vi "AlignDUT_Striptest.vi"(9 "New Sensor?":bool, 10 "ProbeStationControl in":refnum<class "ProbeStationControl.lvclass">) -> (2 "ProbeStationControl in 3":refnum<class "ProbeStationControl.lvclass">)   [LabVIEW 2019]
uses:
  itk-strip-sensor-qc/LabVIEW 2019/InstrControl/ProbeStationControl/ProbeStationControl.lvclass
  <vilib>/userDefined/High Color/IMAQdx.ctl
  <vilib>/vision/driver/NI_Vision_Acquisition_Software.lvlib
  <vilib>/vision/NI_Vision_Development_Module.lvlib
panel:
  out "Average Length Between Fiducials":dbl format="%0.2f"
  in  "Number of Iterations":i32=1
  in  "Sensor Type":string(combo)="ATLAS12R0"
  in  "Second Move OK?":bool
  in  "Second Fiducial OK?":bool
  in  "Second Fiducial in View?":bool
  in  "First Move OK?":bool
  in  "First Fiducial OK?":bool
  out "Pattern Matched Image":T1(plugin-control) caption="Template Image"
  out "Image Out":T1(plugin-control)
  in  "Fiducial 1":bool
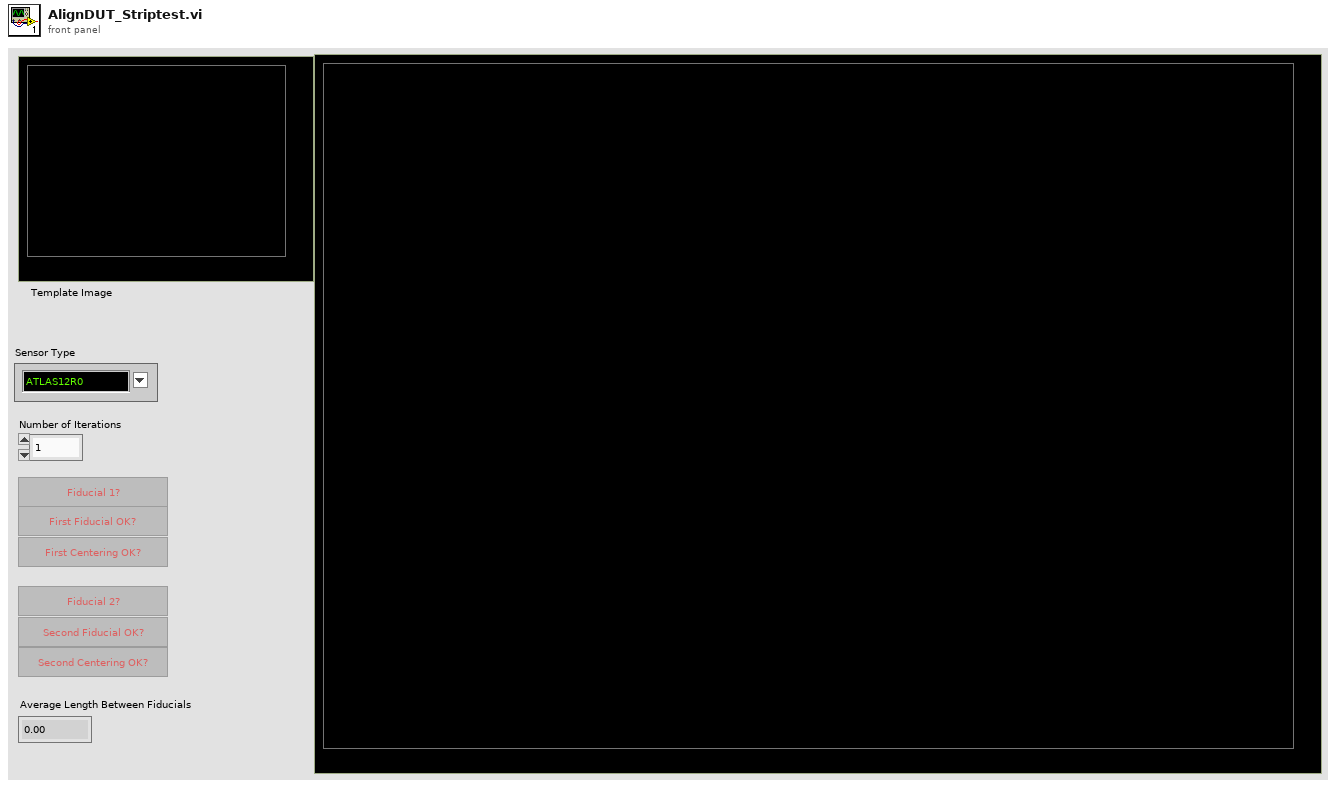
[diagram p1: front panel]
types:
  T1 = typedef "IMAQ Image.ctl" = refnum<image>
  T2 = typedef "IMAQdx.ctl" = refnum<k21>
  T3 = enum8{"Enabled", "Disabled", "Disabled and Grayed Out"}
  T4 = typedef "Image Type" = u32
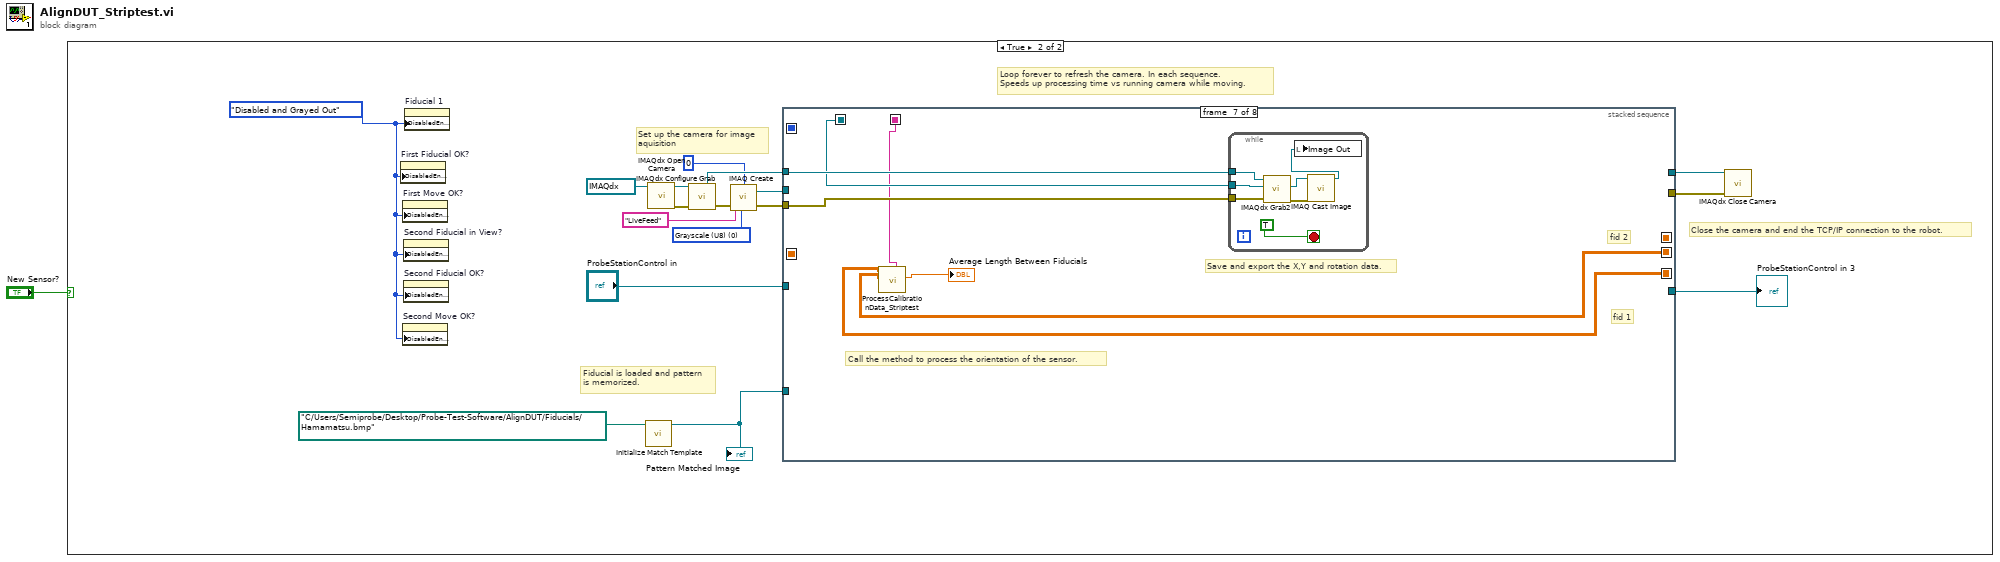
[diagram p0: block diagram]
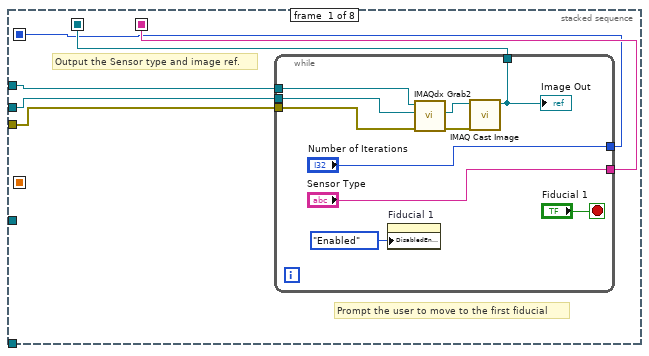
[diagram p3: hidden frame]
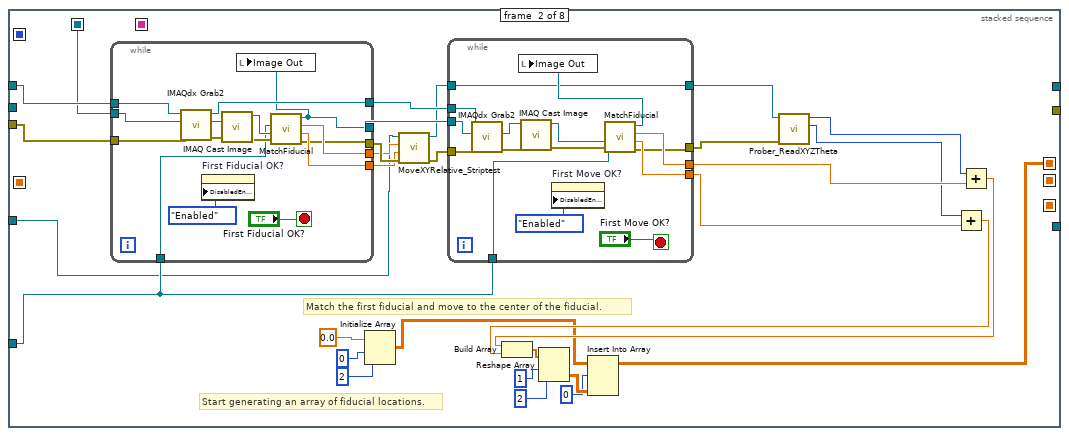
[diagram p4: hidden frame]
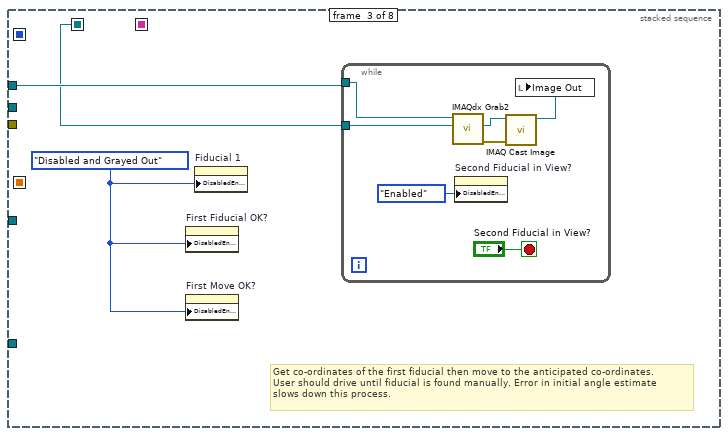
[diagram p5: hidden frame]
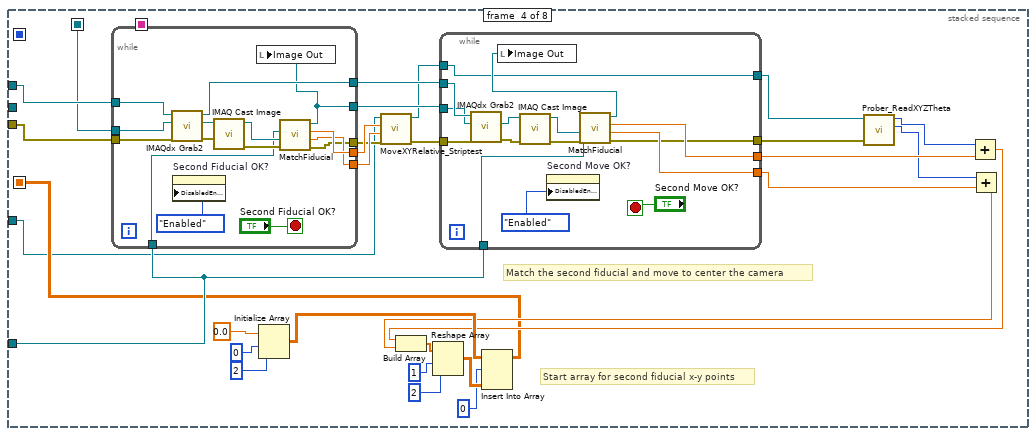
[diagram p6: hidden frame]
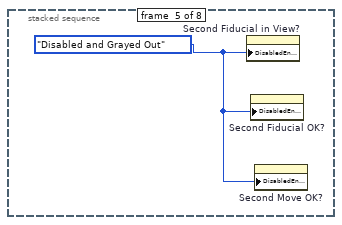
[diagram p7: hidden frame]
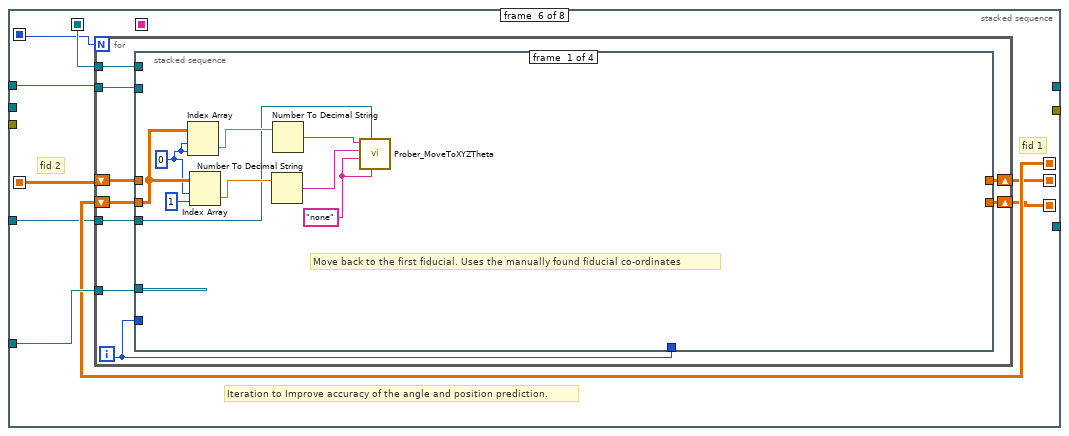
[diagram p8: hidden frame]
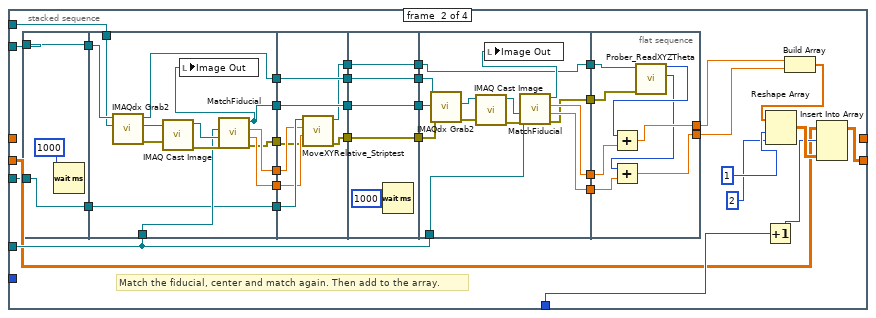
[diagram p9: hidden frame]
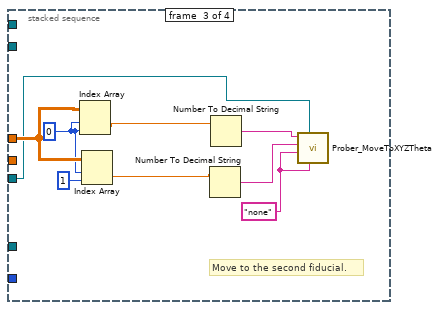
[diagram p10: hidden frame]
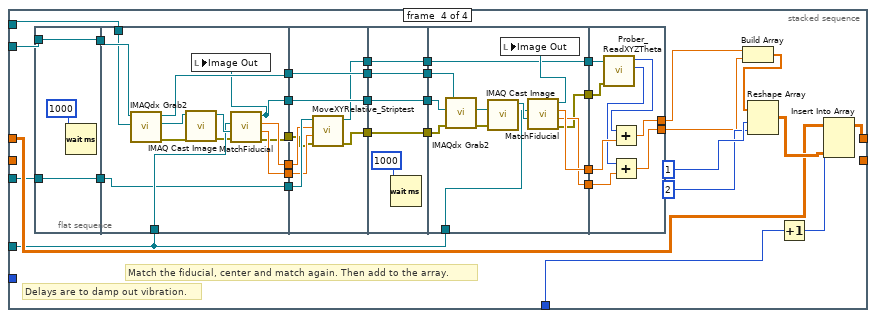
[diagram p11: hidden frame]
diagram:
  n1 = case shown="True" "New Sensor?" {
    frame False {
    }
    frame True {
      w5 = T3."Disabled and Grayed Out" ("Disabled")
      w7 = T4 0 items=["Grayscale (U8)", "Grayscale (I16)", "Grayscale (SGL)", "Complex (CSG)", "RGB (U32)", "HSL (U32)", "RGB (U64)", "Grayscale (U16)"] ("Image Type")
      # "Close the camera and end the TCP/IP connection to the robot."
      # "Fiducial is loaded and pattern\nis memorized."
      # "Loop forever to refresh the camera. In each sequence. \nSpeeds up processing time vs running camera while moving."
      # "Set up the camera for image \naquisition"
      n2 = property on="First Fiducial OK?" class="Bool"("DisabledEnum"=w5) -> ()  [unwired: 2 in, 2 out]
      n3 = property on="First Move OK?" class="Bool"("DisabledEnum"=w5) -> ()  [unwired: 2 in, 2 out]
      n4 = property on="Second Move OK?" class="Bool"("DisabledEnum"=w5) -> ()  [unwired: 2 in, 2 out]
      n5 = property on="Second Fiducial in View?" class="Bool"("DisabledEnum"=w5) -> ()  [unwired: 2 in, 2 out]
      n6 = property on="Second Fiducial OK?" class="Bool"("DisabledEnum"=w5) -> ()  [unwired: 2 in, 2 out]
      n7 = property on="Fiducial 1" class="Bool"("DisabledEnum"=w5) -> ()  [unwired: 2 in, 2 out]
      n8 = call "Initialize Match Template.vi"("base path"=path "C:/Users/Semiprobe/Desktop/Probe-Test-Software/AlignDUT/Fiducials/Hamamatsu.bmp") -> ("Pattern Matched Image"=w10:T1)  [unwired: 10 in]
      "Pattern Matched Image" <- w10
      n9 = call <vilib>:"IMAQdx Open Camera.vi"("Session In"=T2 "cam0") -> ("error out"=w16:errorcluster, "Session Out"=w17:T2)  [unwired: 9 in]
      n10 = call <vilib>:"IMAQdx Configure Grab.vi"("error in"=w16, "Session In"=w17) -> ("error out"=w14:errorcluster, "Session Out"=w13:T2)  [unwired: 8 in]
      n11 = call "IMAQ Create"("Border Size"=0, "Image Name"="LiveFeed", "Image Type"=w7, "error in (no error)"=w14) -> ("New Image"=w12:T1, "error out"=w11:errorcluster)  [unwired: 1 in]
      n12 = stacked-sequence {
        seq-local: [_ _ _ w115 _ _ _ _] -> [_ _ _ _ _ w174 _ _]
        seq-local: [w21 _ _ _ _ _ _ _] -> [_ w59 w96 w130 _ w173 w373 _]
        seq-local: [_ w46 _ _ _ _ _ _] -> [_ _ _ _ _ w170 _ _]
        seq-local: [_ _ _ _ _ w168 _ _] -> [_ _ _ _ _ _ w371 _]
        seq-local: [_ _ _ _ _ w169 _ _] -> [_ _ _ _ _ _ w372 _]
        seq-local: [w20 _ _ _ _ _ _ _] -> [_ _ _ _ _ _ w370 _]
        seq-local: [w19 _ _ _ _ _ _ _] -> [_ _ _ _ _ w167 _ _]
        tunnel: w13 -> [w24 w64 w97 w131 _ w172 w375 w384]
        tunnel: w12 -> [w23 _ _ _ _ _ _ _]
        tunnel: w11 -> [w22 w61 _ w133 _ _ w374 w385]
        tunnel: w10 -> [_ w62 _ w132 _ w171 _ _]
        tunnel: [_ _ _ _ _ _ _ w385] -> w9
        tunnel: [_ _ _ _ _ _ _ w384] -> w8
        tunnel: "ProbeStationControl in" -> [_ w41 _ w110 _ w166 _ w383]
        tunnel: [_ _ _ _ _ _ _ w383] -> w3
        frame #0 {
          # "Output the Sensor type and image ref."
          # "Prompt the user to move to the first fiducial"
          n13 = while {
            tunnel: w24 -> [w33]
            tunnel: w22 -> [w32]
            tunnel: w23 -> [w31]
            tunnel: [w28] -> w21
            tunnel: ["Sensor Type"] -> w20
            tunnel: ["Number of Iterations"] -> w19
            stop <- "Fiducial 1" stop-if-true
            n14 = property on="Fiducial 1" class="Bool"("DisabledEnum"=T3."Enabled" ("Disabled")) -> ()  [unwired: 2 in, 2 out]
            n15 = call <vilib>:"IMAQdx Grab2.vi"("error in"=w32, "Image In"=w31, "Session In"=w33) -> ("error out"=w29:errorcluster, "Image Out"=w30:T1)  [unwired: 5 in, 2 out]
            n16 = call "IMAQ Cast Image"("error in (no error)"=w29, "Image Src"=w30) -> ("Image Dst Out"=w28:T1)  [unwired: 8 in, 1 out]
            "Image Out" <- w28
          }
        }
        frame #1 {
          # "Start generating an array of fiducial locations."
          # "Match the first fiducial and move to the center of the fiducial."
          n17 = while {
            tunnel: [w81] -> w60
            tunnel: [w94] -> w63
            tunnel: [w85] -> w44
            tunnel: w64 -> [w92]
            tunnel: w62 -> [w82]
            tunnel: w61 -> [w87]
            tunnel: [w91] -> w43
            tunnel: [w90] -> w42
            tunnel: w59 -> [w86]
            stop <- "First Fiducial OK?" stop-if-true
            n18 = call <vilib>:"IMAQdx Grab2.vi"("error in"=w87, "Image In"=w86, "Session In"=w92) -> ("error out"=w89:errorcluster, "Image Out"=w88:T1, "Session Out"=w94:T2)  [unwired: 5 in, 1 out]
            n19 = property on="First Fiducial OK?" class="Bool"("DisabledEnum"=T3."Enabled" ("Disabled")) -> ()  [unwired: 2 in, 2 out]
            n20 = call "IMAQ Cast Image"("error in (no error)"=w89, "Image Src"=w88) -> ("error out"=w84:errorcluster, "Image Dst Out"=w83:T1)  [unwired: 8 in]
            n21 = call "MatchFiducial.vi"("error in"=w84, "Image In"=w83, "Template Image"=w82) -> ("error out"=w85:errorcluster, "Y (um)"=w90:dbl, "X (um)"=w91:dbl, "Image Out"=w81:T1)  [unwired: 3 in, 2 out]
            n22 = local write "Image Out"(w81) -> ()
          }
          n23 = Initialize Array(0.0 ("element"), 0 ("dimension size"), 2 ("dimension size")) -> (w47:dbl[][])
          n24 = call "MoveXYRelative_Striptest.vi"("error in (no error)"=w44, "Y_Offset"=w42, "X_Offset"=w43, "ProbeStationControl in"=w41) -> ("error out"=w35:errorcluster, "ProbeStationControl out 2"=w40:refnum<class "ProbeStationControl.lvclass">)  [unwired: 6 in]
          n25 = while {
            tunnel: w63 -> [w78]
            tunnel: w35 -> [w72]
            tunnel: w62 -> [w67]
            tunnel: w60 -> [w73]
            tunnel: [w75] -> w54
            tunnel: [w74] -> w55
            tunnel: [w68] -> w36
            tunnel: w40 -> [w65]
            tunnel: [w65] -> w37
            stop <- "First Move OK?" stop-if-true
            n26 = call <vilib>:"IMAQdx Grab2.vi"("error in"=w72, "Image In"=w73, "Session In"=w78) -> ("error out"=w77:errorcluster, "Image Out"=w76:T1)  [unwired: 5 in, 2 out]
            n27 = call "IMAQ Cast Image"("error in (no error)"=w77, "Image Src"=w76) -> ("error out"=w71:errorcluster, "Image Dst Out"=w70:T1)  [unwired: 8 in]
            n28 = property on="First Move OK?" class="Bool"("DisabledEnum"=T3."Enabled" ("Disabled")) -> ()  [unwired: 2 in, 2 out]
            n29 = call "MatchFiducial.vi"("error in"=w71, "Image In"=w70, "Template Image"=w67) -> ("error out"=w68:errorcluster, "Y (um)"=w75:dbl, "X (um)"=w74:dbl, "Image Out"=w69:T1)  [unwired: 3 in, 2 out]
            n30 = local write "Image Out"(w69) -> ()
          }
          n31 = call-dynamic "Prober_ReadXYZTheta.vi"("error in (no error)"=w36, "ProbeStationControl in"=w37) -> ("Y location [µm]"=w38:i32, "X location [µm]"=w39:i32)  [unwired: 4 in, 4 out]
          n32 = Add(x=w38, y=w54) -> (x+y=w48:dbl)
          n33 = Add(x=w39, y=w55) -> (x+y=w49:dbl)
          n34 = Build Array(w49, w48) -> (w53:dbl[])
          n35 = Reshape Array(w53, 1 ("dimension size"), 2 ("dimension size")) -> (w52:dbl[][])
          n36 = Insert Into Array(array=w47, index (row)=0, new element=w52) -> (w46:dbl[][])  [unwired: 1 in]
        }
        frame #2 {
          w95 = T3."Disabled and Grayed Out" ("Disabled")
          # "Get co-ordinates of the first fiducial then move to the anticipated co-ordinates. \nUser should drive until fiducial is found manually. Error in initial angle estimate \nslows down this process."
          n37 = property on="First Fiducial OK?" class="Bool"("DisabledEnum"=w95) -> ()  [unwired: 2 in, 2 out]
          n38 = property on="First Move OK?" class="Bool"("DisabledEnum"=w95) -> ()  [unwired: 2 in, 2 out]
          n39 = property on="Fiducial 1" class="Bool"("DisabledEnum"=w95) -> ()  [unwired: 2 in, 2 out]
          n40 = while {
            tunnel: w96 -> [w103]
            tunnel: w97 -> [w102]
            stop <- "Second Fiducial in View?" stop-if-true
            n41 = call <vilib>:"IMAQdx Grab2.vi"("Image In"=w103, "Session In"=w102) -> ("error out"=w101:errorcluster, "Image Out"=w100:T1)  [unwired: 6 in, 2 out]
            n42 = property on="Second Fiducial in View?" class="Bool"("DisabledEnum"=T3."Enabled" ("Disabled")) -> ()  [unwired: 2 in, 2 out]
            n43 = call "IMAQ Cast Image"("error in (no error)"=w101, "Image Src"=w100) -> ("Image Dst Out"=w99:T1)  [unwired: 8 in, 1 out]
            n44 = local write "Image Out"(w99) -> ()
          }
        }
        frame #3 {
          # "Start array for second fiducial x-y points"
          # "Match the second fiducial and move to center the camera"
          n45 = while {
            tunnel: [w155] -> w134
            tunnel: [w156] -> w111
            tunnel: w131 -> [w163]
            tunnel: w132 -> [w152]
            tunnel: w133 -> [w157]
            tunnel: w130 -> [w158]
            tunnel: [w162] -> w113
            tunnel: [w161] -> w112
            tunnel: [w151] -> w129
            stop <- "Second Fiducial OK?" stop-if-true
            n46 = call <vilib>:"IMAQdx Grab2.vi"("error in"=w157, "Image In"=w158, "Session In"=w163) -> ("error out"=w160:errorcluster, "Image Out"=w159:T1, "Session Out"=w155:T2)  [unwired: 5 in, 1 out]
            n47 = property on="Second Fiducial OK?" class="Bool"("DisabledEnum"=T3."Enabled" ("Disabled")) -> ()  [unwired: 2 in, 2 out]
            n48 = call "IMAQ Cast Image"("error in (no error)"=w160, "Image Src"=w159) -> ("error out"=w153:errorcluster, "Image Dst Out"=w154:T1)  [unwired: 8 in]
            n49 = call "MatchFiducial.vi"("error in"=w153, "Image In"=w154, "Template Image"=w152) -> ("error out"=w156:errorcluster, "Y (um)"=w161:dbl, "X (um)"=w162:dbl, "Image Out"=w151:T1)  [unwired: 3 in, 2 out]
            n50 = local write "Image Out"(w151) -> ()
          }
          n51 = Initialize Array(0.0 ("element"), 0 ("dimension size"), 2 ("dimension size")) -> (w119:dbl[][])
          n52 = call "MoveXYRelative_Striptest.vi"("error in (no error)"=w111, "Y_Offset"=w112, "X_Offset"=w113, "ProbeStationControl in"=w110) -> ("error out"=w114:errorcluster, "ProbeStationControl out 2"=w109:refnum<class "ProbeStationControl.lvclass">)  [unwired: 6 in]
          n53 = while {
            tunnel: w134 -> [w148]
            tunnel: w114 -> [w142]
            tunnel: w132 -> [w139]
            tunnel: w129 -> [w143]
            tunnel: [w145] -> w128
            tunnel: [w144] -> w127
            tunnel: [w137] -> w106
            tunnel: w109 -> [w135]
            tunnel: [w135] -> w105
            stop <- "Second Move OK?" stop-if-true
            n54 = call <vilib>:"IMAQdx Grab2.vi"("error in"=w142, "Image In"=w143, "Session In"=w148) -> ("error out"=w147:errorcluster, "Image Out"=w146:T1)  [unwired: 5 in, 2 out]
            n55 = call "IMAQ Cast Image"("error in (no error)"=w147, "Image Src"=w146) -> ("error out"=w141:errorcluster, "Image Dst Out"=w140:T1)  [unwired: 8 in]
            n56 = property on="Second Move OK?" class="Bool"("DisabledEnum"=T3."Enabled" ("Disabled")) -> ()  [unwired: 2 in, 2 out]
            n57 = call "MatchFiducial.vi"("error in"=w141, "Image In"=w140, "Template Image"=w139) -> ("error out"=w137:errorcluster, "Y (um)"=w144:dbl, "X (um)"=w145:dbl, "Image Out"=w138:T1)  [unwired: 3 in, 2 out]
            n58 = local write "Image Out"(w138) -> ()
          }
          n59 = call-dynamic "Prober_ReadXYZTheta.vi"("error in (no error)"=w106, "ProbeStationControl in"=w105) -> ("Y location [µm]"=w107:i32, "X location [µm]"=w108:i32)  [unwired: 4 in, 4 out]
          n60 = Add(x=w108, y=w128) -> (x+y=w117:dbl)
          n61 = Add(x=w107, y=w127) -> (x+y=w116:dbl)
          n62 = Build Array(w117, w116) -> (w123:dbl[])
          n63 = Reshape Array(w123, 1 ("dimension size"), 2 ("dimension size")) -> (w122:dbl[][])
          n64 = Insert Into Array(array=w119, index (row)=0, new element=w122) -> (w115:dbl[][])  [unwired: 1 in]
        }
        frame #4 {
          w165 = T3."Disabled and Grayed Out" ("Disabled")
          n65 = property on="Second Fiducial in View?" class="Bool"("DisabledEnum"=w165) -> ()  [unwired: 2 in, 2 out]
          n66 = property on="Second Fiducial OK?" class="Bool"("DisabledEnum"=w165) -> ()  [unwired: 2 in, 2 out]
          n67 = property on="Second Move OK?" class="Bool"("DisabledEnum"=w165) -> ()  [unwired: 2 in, 2 out]
        }
        frame #5 {
          # "fid 1"
          # "fid 2"
          # "Iteration to Improve accuracy of the angle and position prediction."
          n68 = for {
            N: w167 -> [_]
            tunnel: w173 -> [w181]
            tunnel: w172 -> [w180]
            tunnel: w171 -> [w182]
            shift-right: [w177] -> w168
            shift-left: w174 -> [w183]
            shift-right: [w178] -> w169
            shift-left: w170 -> [w179]
            tunnel: w166 -> [w175]
            i -> [w176]
            n69 = stacked-sequence {
              tunnel: w183 -> [_ _ w284 w304]
              tunnel: w182 -> [_ w224 _ w294]
              tunnel: w176 -> [_ w216 _ w307]
              tunnel: w181 -> [_ w213 _ w305]
              tunnel: w180 -> [_ w214 _ w306]
              tunnel: w179 -> [w191 w212 _ _]
              tunnel: [_ w211 _ _] -> w178
              tunnel: [_ _ _ w303] -> w177
              tunnel: w176 -> [_ _ _ _]
              tunnel: w175 -> [w184 w197 w279 w290]
              frame #0 {
                w185 = "none" ("Z location [µm]")
                w190 = 0 ("index (row)")
                # "Move back to the first fiducial. Uses the manually found fiducial co-ordinates"
                n70 = Index Array(array=w191, index (row)=w190, index (col)=w190) -> (element=w189:dbl)
                n71 = Index Array(array=w191, index (row)=w190, index (col)=1) -> (element=w188:dbl)
                n72 = Number To Decimal String(number=w188) -> (decimal integer string=w186:string)  [unwired: 1 in]
                n73 = Number To Decimal String(number=w189) -> (decimal integer string=w187:string)  [unwired: 1 in]
                n74 = call-dynamic "Prober_MoveToXYZTheta.vi"("Theta location [mdeg]"=w185, "ProbeStationControl in"=w184, "Z location [µm]"=w185, "Y location [µm]"=w186, "X location [µm]"=w187) -> ()  [unwired: 4 in, 3 out]
              }
              frame #1 {
                # "Match the fiducial, center and match again. Then add to the array."
                n75 = flat-sequence {
                  tunnel: w214 -> [w229]
                  tunnel: [w229] -> w202
                  tunnel: [w227] -> w198
                  tunnel: w197 -> [w227]
                  tunnel: w224 -> [w232]
                  tunnel: [w234] -> w226
                  tunnel: [w239] -> w225
                  tunnel: w213 -> [w236]
                  tunnel: [w238] -> w210
                  tunnel: [w237] -> w209
                  tunnel: w202 -> [w240]
                  tunnel: [w231] -> w201
                  tunnel: w198 -> [w230]
                  tunnel: [w230] -> w196
                  tunnel: w226 -> [w244]
                  tunnel: w225 -> [w250]
                  tunnel: [w250] -> w208
                  tunnel: [w249] -> w206
                  tunnel: [w243] -> w204
                  tunnel: w210 -> [w247]
                  tunnel: w209 -> [w246]
                  tunnel: w201 -> [w249]
                  tunnel: w196 -> [w248]
                  tunnel: [w245] -> w195
                  tunnel: w208 -> [w255]
                  tunnel: [w255] -> w207
                  tunnel: w206 -> [w254]
                  tunnel: [w254] -> w205
                  tunnel: w204 -> [w253]
                  tunnel: [w253] -> w203
                  tunnel: w195 -> [w251]
                  tunnel: [w251] -> w193
                  tunnel: w207 -> [w266]
                  tunnel: w205 -> [w258]
                  tunnel: w203 -> [w263]
                  tunnel: w224 -> [w260]
                  tunnel: [w262] -> w223
                  tunnel: [w265] -> w221
                  tunnel: [w264] -> w220
                  tunnel: [w257] -> w194
                  tunnel: w193 -> [w257]
                  tunnel: w223 -> [w271]
                  tunnel: w221 -> [w276]
                  tunnel: w220 -> [w275]
                  tunnel: [w274] -> w200
                  tunnel: [w273] -> w199
                  tunnel: w194 -> [w272]
                  frame #0 {
                    n76 = Wait (ms)(milliseconds to wait=u32 1000) -> ()  [unwired: 1 out]
                  }
                  frame #1 {
                    n77 = call <vilib>:"IMAQdx Grab2.vi"("Image In"=w236, "Session In"=w240) -> ("error out"=w242:errorcluster, "Image Out"=w241:T1, "Session Out"=w239:T2)  [unwired: 6 in, 1 out]
                    n78 = call "IMAQ Cast Image"("error in (no error)"=w242, "Image Src"=w241) -> ("error out"=w235:errorcluster, "Image Dst Out"=w233:T1)  [unwired: 8 in]
                    n79 = call "MatchFiducial.vi"("error in"=w235, "Image In"=w233, "Template Image"=w232) -> ("error out"=w234:errorcluster, "Y (um)"=w237:dbl, "X (um)"=w238:dbl, "Image Out"=w231:T1)  [unwired: 3 in, 2 out]
                    n80 = local write "Image Out"(w231) -> ()
                  }
                  frame #2 {
                    n81 = call "MoveXYRelative_Striptest.vi"("error in (no error)"=w244, "Y_Offset"=w246, "X_Offset"=w247, "ProbeStationControl in"=w248) -> ("error out"=w243:errorcluster, "ProbeStationControl out 2"=w245:refnum<class "ProbeStationControl.lvclass">)  [unwired: 6 in]
                  }
                  frame #3 {
                    n82 = Wait (ms)(milliseconds to wait=u32 1000) -> ()  [unwired: 1 out]
                  }
                  frame #4 {
                    n83 = call <vilib>:"IMAQdx Grab2.vi"("error in"=w263, "Image In"=w258, "Session In"=w266) -> ("error out"=w267:errorcluster, "Image Out"=w268:T1)  [unwired: 5 in, 2 out]
                    n84 = call "IMAQ Cast Image"("error in (no error)"=w267, "Image Src"=w268) -> ("error out"=w256:errorcluster, "Image Dst Out"=w261:T1)  [unwired: 8 in]
                    n85 = call "MatchFiducial.vi"("error in"=w256, "Image In"=w261, "Template Image"=w260) -> ("error out"=w262:errorcluster, "Y (um)"=w264:dbl, "X (um)"=w265:dbl, "Image Out"=w259:T1)  [unwired: 3 in, 2 out]
                    n86 = local write "Image Out"(w259) -> ()
                  }
                  frame #5 {
                    n87 = call-dynamic "Prober_ReadXYZTheta.vi"("error in (no error)"=w271, "ProbeStationControl in"=w272) -> ("Y location [µm]"=w269:i32, "X location [µm]"=w270:i32)  [unwired: 4 in, 4 out]
                    n88 = Add(x=w270, y=w276) -> (x+y=w274:dbl)
                    n89 = Add(x=w269, y=w275) -> (x+y=w273:dbl)
                  }
                }
                n90 = Increment(x=w216) -> (x+1=w215:i32)
                n91 = Build Array(w200, w199) -> (w219:dbl[])
                n92 = Reshape Array(w219, 1 ("dimension size"), 2 ("dimension size")) -> (w222:dbl[][])
                n93 = Insert Into Array(array=w212, index (row)=w215, new element=w222) -> (w211:dbl[][])  [unwired: 1 in]
              }
              frame #2 {
                w280 = "none" ("Z location [µm]")
                w283 = 0 ("index (row)")
                # "Move to the second fiducial."
                n94 = Index Array(array=w284, index (row)=w283, index (col)=w283) -> (element=w277:dbl)
                n95 = Index Array(array=w284, index (row)=w283, index (col)=1) -> (element=w278:dbl)
                n96 = Number To Decimal String(number=w278) -> (decimal integer string=w281:string)  [unwired: 1 in]
                n97 = Number To Decimal String(number=w277) -> (decimal integer string=w282:string)  [unwired: 1 in]
                n98 = call-dynamic "Prober_MoveToXYZTheta.vi"("Theta location [mdeg]"=w280, "ProbeStationControl in"=w279, "Z location [µm]"=w280, "Y location [µm]"=w281, "X location [µm]"=w282) -> ()  [unwired: 4 in, 3 out]
              }
              frame #3 {
                # "Delays are to damp out vibration."
                # "Match the fiducial, center and match again. Then add to the array."
                n99 = flat-sequence {
                  tunnel: w306 -> [w322]
                  tunnel: [w322] -> w295
                  tunnel: [w320] -> w291
                  tunnel: w290 -> [w320]
                  tunnel: w294 -> [w327]
                  tunnel: [w332] -> w319
                  tunnel: [w324] -> w318
                  tunnel: [w329] -> w317
                  tunnel: [w326] -> w316
                  tunnel: w305 -> [w330]
                  tunnel: [w331] -> w302
                  tunnel: w295 -> [w333]
                  tunnel: w291 -> [w323]
                  tunnel: [w323] -> w289
                  tunnel: w319 -> [w339]
                  tunnel: w318 -> [w338]
                  tunnel: w317 -> [w343]
                  tunnel: w316 -> [w342]
                  tunnel: [w343] -> w301
                  tunnel: [w342] -> w299
                  tunnel: [w337] -> w297
                  tunnel: w302 -> [w340]
                  tunnel: w289 -> [w341]
                  tunnel: [w336] -> w288
                  tunnel: w301 -> [w348]
                  tunnel: [w348] -> w300
                  tunnel: w299 -> [w347]
                  tunnel: [w347] -> w298
                  tunnel: w297 -> [w346]
                  tunnel: [w346] -> w296
                  tunnel: w288 -> [w344]
                  tunnel: [w344] -> w287
                  tunnel: w300 -> [w358]
                  tunnel: w298 -> [w355]
                  tunnel: w296 -> [w354]
                  tunnel: w294 -> [w352]
                  tunnel: [w350] -> w315
                  tunnel: [w357] -> w314
                  tunnel: [w356] -> w313
                  tunnel: w287 -> [w349]
                  tunnel: [w349] -> w286
                  tunnel: w315 -> [w361]
                  tunnel: w314 -> [w368]
                  tunnel: w313 -> [w367]
                  tunnel: [w366] -> w293
                  tunnel: [w365] -> w292
                  tunnel: w286 -> [w362]
                  frame #0 {
                    n100 = Wait (ms)(milliseconds to wait=u32 1000) -> ()  [unwired: 1 out]
                  }
                  frame #1 {
                    n101 = call <vilib>:"IMAQdx Grab2.vi"("Image In"=w330, "Session In"=w333) -> ("error out"=w335:errorcluster, "Image Out"=w334:T1, "Session Out"=w329:T2)  [unwired: 6 in, 1 out]
                    n102 = call "IMAQ Cast Image"("error in (no error)"=w335, "Image Src"=w334) -> ("error out"=w325:errorcluster, "Image Dst Out"=w328:T1)  [unwired: 8 in]
                    n103 = call "MatchFiducial.vi"("error in"=w325, "Image In"=w328, "Template Image"=w327) -> ("error out"=w324:errorcluster, "Y (um)"=w332:dbl, "X (um)"=w331:dbl, "Image Out"=w326:T1)  [unwired: 3 in, 2 out]
                    n104 = local write "Image Out"(w326) -> ()
                  }
                  frame #2 {
                    n105 = call "MoveXYRelative_Striptest.vi"("error in (no error)"=w338, "Y_Offset"=w339, "X_Offset"=w340, "ProbeStationControl in"=w341) -> ("error out"=w337:errorcluster, "ProbeStationControl out 2"=w336:refnum<class "ProbeStationControl.lvclass">)  [unwired: 6 in]
                  }
                  frame #3 {
                    n106 = Wait (ms)(milliseconds to wait=u32 1000) -> ()  [unwired: 1 out]
                  }
                  frame #4 {
                    n107 = call <vilib>:"IMAQdx Grab2.vi"("error in"=w354, "Image In"=w355, "Session In"=w358) -> ("error out"=w359:errorcluster, "Image Out"=w360:T1)  [unwired: 5 in, 2 out]
                    n108 = call "IMAQ Cast Image"("error in (no error)"=w359, "Image Src"=w360) -> ("Image Dst Out"=w353:T1)  [unwired: 8 in, 1 out]
                    n109 = call "MatchFiducial.vi"("Image In"=w353, "Template Image"=w352) -> ("error out"=w350:errorcluster, "Y (um)"=w356:dbl, "X (um)"=w357:dbl, "Image Out"=w351:T1)  [unwired: 4 in, 2 out]
                    n110 = local write "Image Out"(w351) -> ()
                  }
                  frame #5 {
                    n111 = call-dynamic "Prober_ReadXYZTheta.vi"("error in (no error)"=w361, "ProbeStationControl in"=w362) -> ("Y location [µm]"=w363:i32, "X location [µm]"=w364:i32)  [unwired: 4 in, 4 out]
                    n112 = Add(x=w364, y=w368) -> (x+y=w366:dbl)
                    n113 = Add(x=w363, y=w367) -> (x+y=w365:dbl)
                  }
                }
                n114 = Build Array(w293, w292) -> (w311:dbl[])
                n115 = Reshape Array(w311, 1 ("dimension size"), 2 ("dimension size")) -> (w312:dbl[][])
                n116 = Increment(x=w307) -> (x+1=w308:i32)
                n117 = Insert Into Array(array=w304, index (row)=w308, new element=w312) -> (w303:dbl[][])  [unwired: 1 in]
              }
            }
          }
        }
        frame #6 {
          # "Call the method to process the orientation of the sensor."
          # "fid 2"
          # "fid 1"
          # "Save and export the X,Y and rotation data."
          n118 = call "ProcessCalibrationData_Striptest.vi"("Sensor Type"=w370, "Fiducial 2"=w371, "Fiducial 1"=w372) -> ("Avg Length"=→"Average Length Between Fiducials":dbl)  [unwired: 8 in]
          n119 = while {
            tunnel: w375 -> [w382]
            tunnel: w373 -> [w381]
            tunnel: w374 -> [w380]
            stop <- TRUE ("Computation OK?") stop-if-true
            n120 = call <vilib>:"IMAQdx Grab2.vi"("error in"=w380, "Image In"=w381, "Session In"=w382) -> ("error out"=w379:errorcluster, "Image Out"=w378:T1)  [unwired: 5 in, 2 out]
            n121 = call "IMAQ Cast Image"("error in (no error)"=w379, "Image Src"=w378) -> ("Image Dst Out"=w377:T1)  [unwired: 8 in, 1 out]
            n122 = local write "Image Out"(w377) -> ()
          }
        }
        frame #7 {
          # "Close connections"
        }
      }
      "ProbeStationControl in 3" <- w3
      n123 = call <vilib>:"IMAQdx Close Camera.vi"("error in"=w9, "Session In"=w8) -> ()  [unwired: 9 in, 1 out]
    }
  }
